vi "log_data.vi"(0 "Data":u64, 5 "File Name":string, 7 "File size(kb)":i64, 11 "error in":errorcluster) -> (4 "File Name out":string, 6 "Stop_logging":bool, 15 "error out":errorcluster)   [LabVIEW 2023, in "task-1.lvlib"]
uses:
  <vilib>/Utility/error.llb/DialogType.ctl
  <vilib>/Utility/error.llb/Trim Whitespace One-Sided.vi
  <vilib>/regexp/Match Regular Expression.xnode
  task-1.lvlib
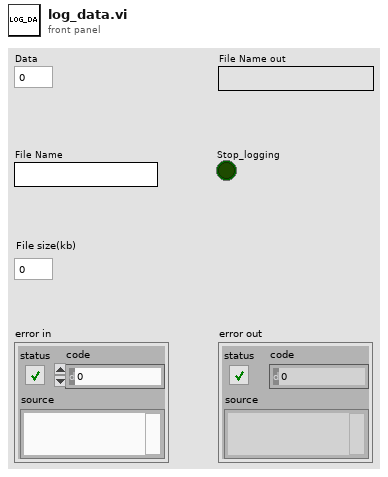
[diagram p1: front panel]
types:
  T1 = enum16{"open", "replace", "create", "open or create", "replace or create", "replace or create with confirmation"}
  T2 = typedef "DialogType.ctl" = u16
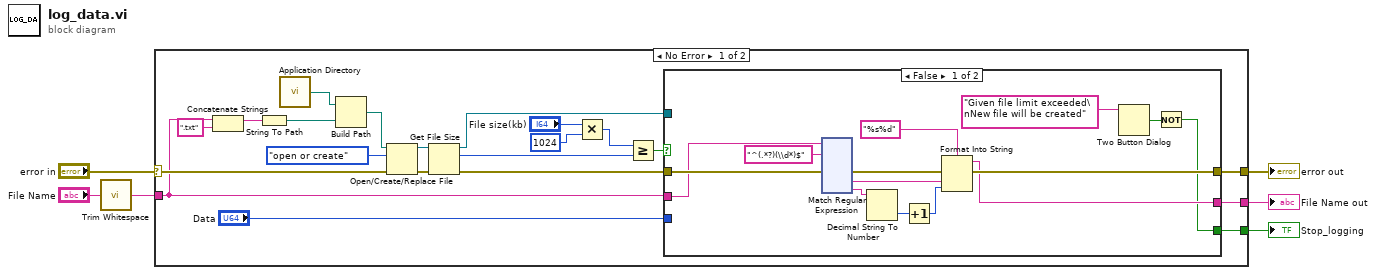
[diagram p0: block diagram]
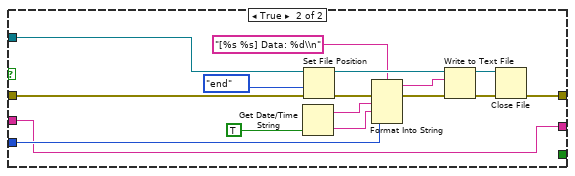
[diagram p2: hidden frame]
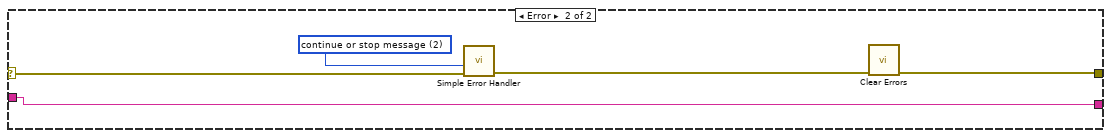
[diagram p3: hidden frame]
diagram:
  n1 = call <vilib>:"Trim Whitespace.vi"("string"="File Name") -> ("trimmed string"=w2:string)  [unwired: 1 in]
  n2 = case shown="No Error" "error in" {
    selector: "error in" -> [w24 w182]
    tunnel: [w17 w180] -> w5
    tunnel: [w11 w178] -> w4
    tunnel: w2 -> [w10 w178]
    tunnel: [w7 _] -> w1
    frame No Error {
      n3 = Concatenate Strings(w10, ".txt" ("string")) -> (w9:string)
      n4 = String To Path(string=w9) -> (path=w21:path)
      n5 = call <vilib>:"Application Directory.vi"() -> ("Application Directory"=w27:path)
      n6 = Build Path(base path=w27, name or relative path=w21) -> (appended path=w26:path)
      n7 = Open/Create/Replace File(file path (use dialog)=w26, error in=w24, operation (0:open)=T1."open or create") -> (refnum out=w23:refnum<file>, error out=w22:errorcluster)  [unwired: 3 in, 1 out]
      n8 = Get File Size(file=w23, error in=w22) -> (refnum out=w16:refnum<file>, size (in bytes)=w20:i64, 0:w15:errorcluster)
      n9 = Multiply(x="File size(kb)", y=i64 1024) -> (x*y=w14:i64)
      n10 = Greater Or Equal?(x=w14, y=w20) -> (x >= y?=w18:bool)
      n11 = case shown="False" w18 {
        tunnel: w15 -> [w36 w177]
        tunnel: [w39 w165] -> w17
        tunnel: w16 -> [_ w173]
        tunnel: "Data" -> [_ w163]
        tunnel: w10 -> [w34 w162]
        tunnel: [w37 w162] -> w11
        tunnel: [w29 _] -> w7
        frame False {
          n12 = xnode "Match Regular Expression"("input string"=w34, "regular expression"="^(.*?)(\\d*)$", "error in"=w36) -> ("error out"=w35:errorcluster, "submatch 1"=w28:string, "submatch 2"=w32:string)  [unwired: 3 in, 4 out]
          n13 = Decimal String To Number(string=w32) -> (number=w31:i32)  [unwired: 2 in, 1 out]
          n14 = Increment(x=w31) -> (x+1=w30:i32)
          n15 = Format Into String(format string="%s%d", error in=w35, w28, w30) -> (resulting string=w37:string, error out=w39:errorcluster)  [unwired: 1 in]
          n16 = Two Button Dialog(message="Given file limit exceeded\nNew file will be created") -> (T button?=w40:bool)  [unwired: 2 in]
          n17 = Not(x=w40) -> (.not. x?=w29:bool)
        }
        frame True {
          n18 = Get Date/Time String(want seconds? (F)=TRUE) -> (date string=w169:string, time string=w168:string)  [unwired: 2 in]
          n19 = Set File Position(refnum=w173, from (0:start)=enum16{"start", "end", "current"}."end", error in=w177) -> (refnum out=w174:refnum<file>, error out=w176:errorcluster)  [unwired: 1 in]
          n20 = Format Into String(format string="[%s %s] Data: %d\\n", error in=w176, w169, w168, w163) -> (resulting string=w166:string, error out=w171:errorcluster)  [unwired: 1 in]
          n21 = Write to Text File(file (use dialog)=w174, text=w166, error in=w171) -> (refnum out=w164:refnum<file>, error out=w175:errorcluster)  [unwired: 1 in, 1 out]
          n22 = Close File(refnum=w164, error in=w175) -> (error out=w165:errorcluster)  [unwired: 1 out]
        }
      }
    }
    frame Error {
      w179 = T2 2 items=["no dialog", "OK message", "continue or stop message", "OK message + warnings", "continue/stop + warnings"] ("type of dialog (OK msg:1)")
      n23 = call <vilib>:"Simple Error Handler.vi"("type of dialog (OK msg:1)"=w179, "error in (no error)"=w182) -> ("error out"=w181:errorcluster)  [unwired: 3 in, 4 out]
      n24 = call <vilib>:"Clear Errors.vi"("error in (no error)"=w181) -> ("error out"=w180:errorcluster)  [unwired: 5 in, 1 out]
    }
  }
  "error out" <- w5
  "File Name out" <- w4
  "Stop_logging" <- w1
